vi "Third Power Control.vi"(11 "upper limit":dbl) -> (3 "Numeric":dbl)   [LabVIEW 2017]
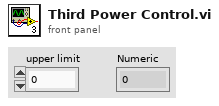
[diagram p1: front panel]
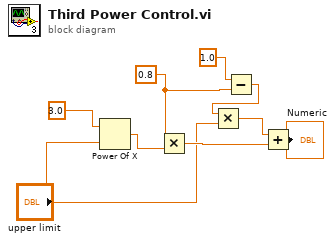
[diagram p0: block diagram]
diagram:
  w9 = 0.8
  n1 = Power Of X(1:"upper limit", 2:3.0) -> (0:w2:dbl)
  n2 = Multiply(x=w9, y=w2) -> (x*y=w8:dbl)
  n3 = Subtract(x=1.0, y=w9) -> (x-y=w4:dbl)
  n4 = Multiply(x=w4, y="upper limit") -> (x*y=w7:dbl)
  n5 = Add(x=w7, y=w8) -> (x+y=→"Numeric":dbl)
